vi "AM Stop.vi"(8 "error in (no error)":errorcluster, 10 "Message Queues out":T1, 11 "Data Cluster":T2 {"PS Measure Plan" items=["Pretreatment settings (PS)", "Linear Sweep Voltammetry (LSV)", "Differential Pulse Voltammetry (DPV)", "Cyclic Voltammetry (CV)", "Chronoamperometry (CA)", "Chronopotentiometry (CP)", "El Imp Spectroscopy (EIS)"]; "System Preset"."Test Configuration"."SP List" format="%#.1g"}) -> (0 "error out":errorcluster, 3 "Data Cluster out":T2 {"PS Measure Plan" items=["Pretreatment settings (PS)", "Linear Sweep Voltammetry (LSV)", "Differential Pulse Voltammetry (DPV)", "Cyclic Voltammetry (CV)", "Chronoamperometry (CA)", "Chronopotentiometry (CP)", "El Imp Spectroscopy (EIS)"]; "System Preset"."Test Configuration"."SP List" format="%#.1g"})   [LabVIEW 2020, in "Test Driver.lvlib"]
uses:
  Test Driver.lvlib
  Test Driver Configuration.ctl
  support/Message Queue/Message Cluster.ctl
  System Preset.ctl
  Test Type.ctl
  support/Message Queue/All Message Queues.ctl
  support/Message Queue/Enqueue Message (Single).vi
  support/Message Queue/Message Queue.lvlib
panel:
  # "X"
  # "Y"
  # "Cycles"
  # "Point Delay"
  # "Up"
  # "Down"
  # "Z Axes"
  # "#C"
  # "In"
  # "Out"
  # "Cleaning [sec]"
  # "X"
  # "Y"
  # "Cycles"
  # "Point Delay"
  # "Up"
  # "Down"
  # "Z Axes"
  # "#C"
  # "In"
  # "Out"
  # "Cleaning [sec]"
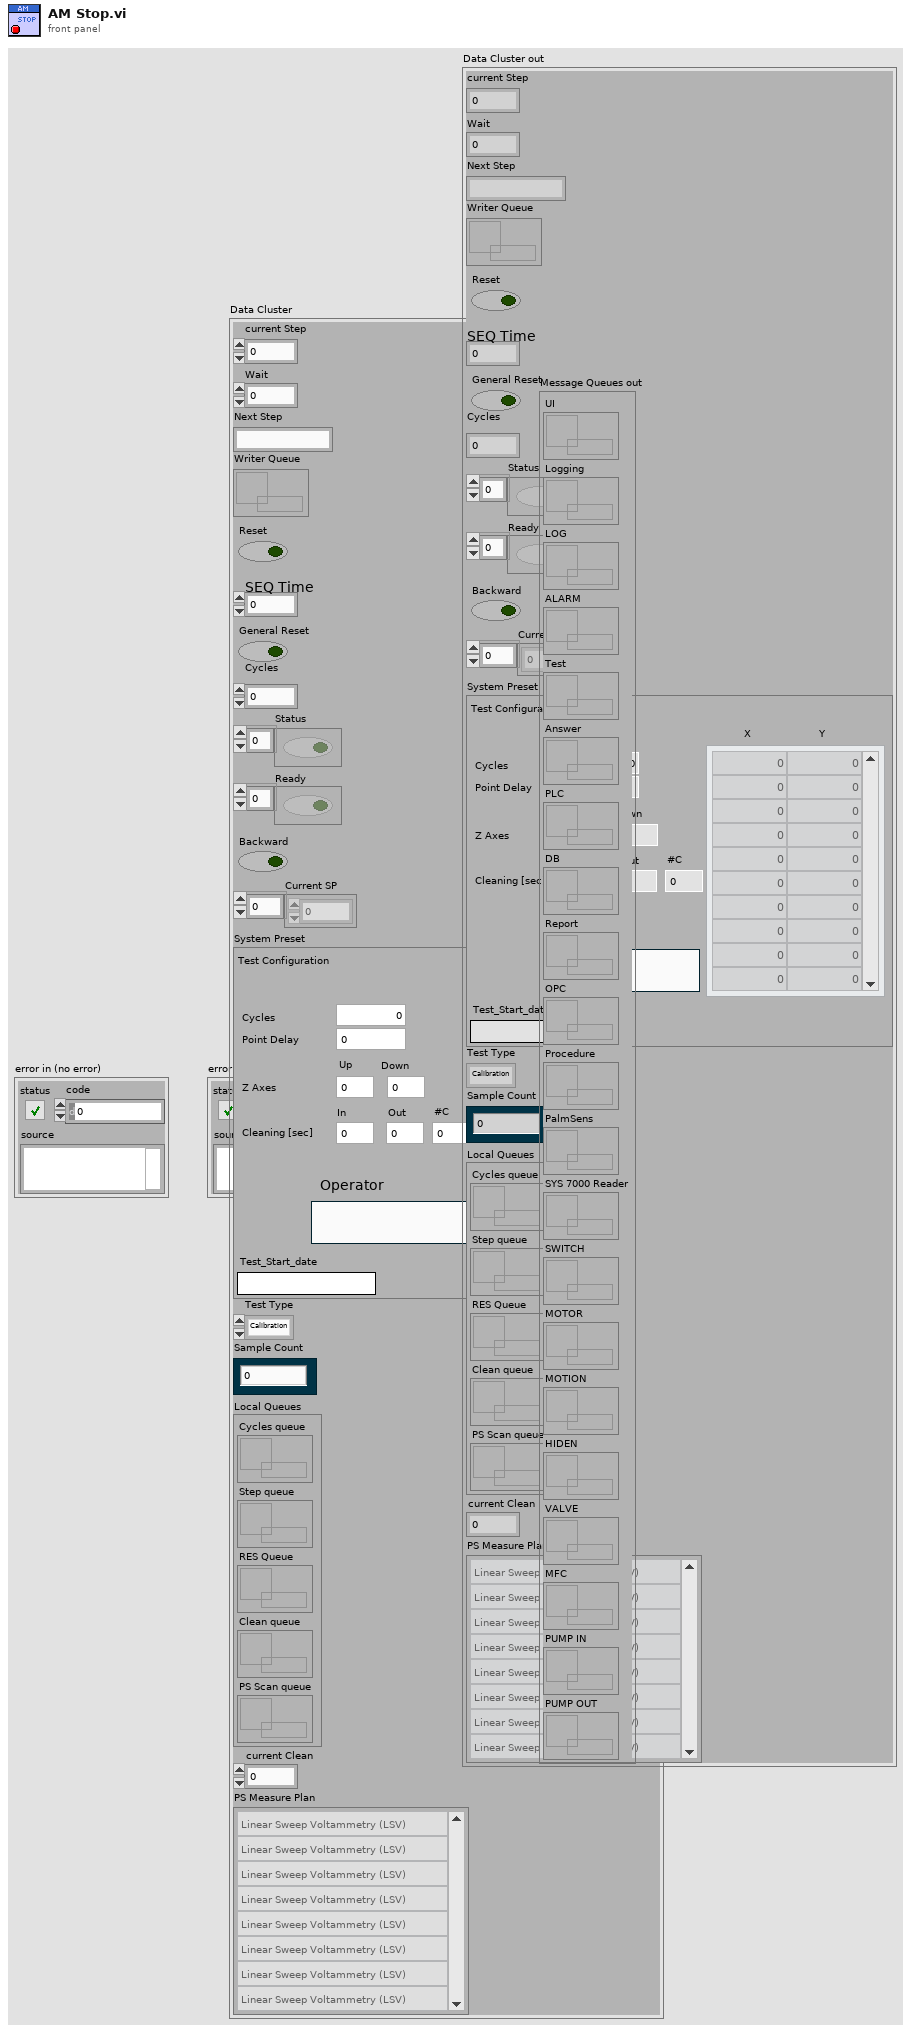
[diagram p1: front panel]
types:
  T1 = typedef "Message Queue.lvlib/All Message Queues.ctl" = cluster{"UI":refnum<queue>, "Logging":refnum<queue>, "LOG":refnum<queue>, "ALARM":refnum<queue>, "Test":refnum<queue>, "Answer":refnum<queue>, "PLC":refnum<queue>, "DB":refnum<queue>, "Report":refnum<queue>, "OPC":refnum<queue>, "Procedure":refnum<queue>, "PalmSens":refnum<queue>, "SYS 7000 Reader":refnum<queue>, "SWITCH":refnum<queue>, "MOTOR":refnum<queue>, "MOTION":refnum<queue>, "HIDEN":refnum<queue>, "VALVE":refnum<queue>, "MFC":refnum<queue>, "PUMP IN":refnum<queue>, "PUMP OUT":refnum<queue>}
  T2 = typedef "Test Driver.lvlib/Test Driver Configuration.ctl" = cluster{"current Step":i32, "Wait":dbl, "Next Step":string, "Writer Queue":refnum<queue>, "Reset":bool, "SEQ Time":i32, "General Reset":bool, "Cycles":i32, "Status":bool[], "Ready":bool[], "Backward":bool, "Current SP":dbl[], "System Preset":T3, "Test Type":T4, "Sample Count":i32, "Local Queues":cluster{"Cycles queue":refnum<queue>, "Step queue":refnum<queue>, "RES Queue":refnum<queue>, "Clean queue":refnum<queue>, "PS Scan queue":refnum<queue>}, "current Clean":i32, "PS Measure Plan":u16[]}
  T3 = typedef "System Preset.ctl" = cluster{"Test Configuration":cluster{"Cycles":i32, "Z Up":dbl, "SP List":dbl[][], "Operator":string, "Point Delay":i32, "Z Up 2":dbl, "Cleaning In":dbl, "Cleaning Out":dbl, "Cleaning Cycles":i32}, "Test_Start_date":string}
  T4 = typedef "Test Driver.lvlib/Test Type.ctl" = enum16{"Calibration", "Test"}
  T5 = typedef "Message Queue.lvlib/Message Cluster.ctl" = cluster{"Message":string, "Message Data":variant}
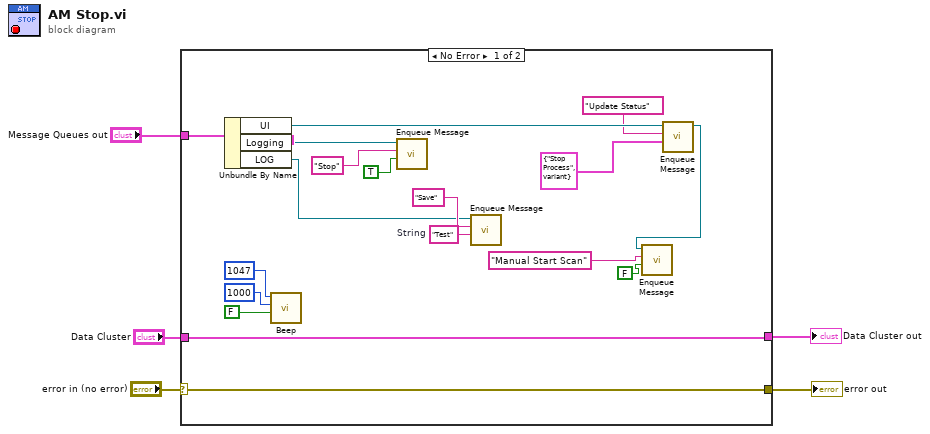
[diagram p0: block diagram]
diagram:
  n1 = case shown="No Error" "error in (no error)" {
    selector: "error in (no error)" -> [w23 w24]
    tunnel: [w18 w25] -> w4
    tunnel: "Data Cluster" -> [w18 w25]
    tunnel: [w23 w24] -> w3
    tunnel: "Message Queues out" -> [w22 _]
    frame No Error {
      w9 = "Test"  # String
      n2 = Unbundle By Name(w22) -> ("UI"=w15:refnum<queue>, "Logging"=w16:refnum<queue>, "LOG"=w10:refnum<queue>)
      n3 = call <vilib>:"Beep.vi"("use system alert? (T)"=FALSE, "duration (msec)"=u32 1000, "frequency (Hz)"=u32 1047) -> ()  [unwired: 9 in]
      n4 = call-poly "Enqueue Message.vi"("Message Data"=TRUE, "Message"="Stop", "Message Queue"=w16) -> ()  [unwired: 7 in, 2 out]
      n5 = call-poly "Enqueue Message.vi"("Message Data"=w9, "Message"="Save" ("Main CMD"), "Message Queue"=w10) -> ()  [unwired: 7 in, 2 out]
      n6 = call-poly "Enqueue Message.vi"("Message Data"=T5 {"Message"="Stop Process", "Message Data"=variant} ("Message Cluster"), "Message"="Update Status", "Message Queue"=w15) -> ("dup Message Queue"=w6:refnum<queue>)  [unwired: 7 in, 1 out]
      n7 = call-poly "Enqueue Message.vi"("Message Data"=FALSE, "Message"="Manual Start Scan", "Message Queue"=w6) -> ()  [unwired: 7 in, 2 out]
    }
    frame Error {
    }
  }
  "error out" <- w3
  "Data Cluster out" <- w4
